vi "input.vi"(8 "error in":errorcluster, 10 "data table in":T1, 11 "io runtime in":refnum<class "io runtime.lvclass">) -> (0 "error out":errorcluster, 2 "data table out":T1, 3 "io runtime out":refnum<class "io runtime.lvclass">)   [LabVIEW 2015, in "io runtime.lvclass"]
doc: "Provides an interface for reading data from a module at runtime. While this interface performs no operations, a child should provide an override which may read from any open sessions, references, or interfaces."
uses:
  io runtime.lvclass
  <vilib>/NI/Tag Bus/table/data table.ctl
  io runtime.lvclass/io runtime.ctl
  FXP I_20_5.ctl
  FXP I_24_5.ctl
  FXP I_24_10.ctl
  <vilib>/NI/Tag Bus/table/data polymorphs/write many/write Doubles.vi
  <vilib>/NI/Tag Bus/table/data polymorphs/write many/write Singles.vi
  <vilib>/NI/Tag Bus/table/data polymorphs/write many/write I64s.vi
  <vilib>/NI/Tag Bus/table/data polymorphs/write many/write I32s.vi
  <vilib>/NI/Tag Bus/table/data polymorphs/write many/write I16s.vi
  <vilib>/NI/Tag Bus/table/data polymorphs/write many/write I8s.vi
  <vilib>/NI/Tag Bus/table/data polymorphs/write many/write U64s.vi
  <vilib>/NI/Tag Bus/table/data polymorphs/write many/write U32s.vi
  <vilib>/NI/Tag Bus/table/data polymorphs/write many/write U16s.vi
  <vilib>/NI/Tag Bus/table/data polymorphs/write many/write U8s.vi
  <vilib>/NI/Tag Bus/table/data polymorphs/write many/write Booleans.vi
  <vilib>/NI/Tag Bus/table/data polymorphs/write one/write Array of Double.vi
  <vilib>/NI/Tag Bus/table/data polymorphs/write one/write Array of Single.vi
  <vilib>/NI/Tag Bus/table/data polymorphs/write one/write Array of I64.vi
  <vilib>/NI/Tag Bus/table/data polymorphs/write one/write Array of I32.vi
  <vilib>/NI/Tag Bus/table/data polymorphs/write one/write Array of I16.vi
  <vilib>/NI/Tag Bus/table/data polymorphs/write one/write Array of I8.vi
  <vilib>/NI/Tag Bus/table/data polymorphs/write one/write Array of U64.vi
  <vilib>/NI/Tag Bus/table/data polymorphs/write one/write Array of U32.vi
  <vilib>/NI/Tag Bus/table/data polymorphs/write one/write Array of U16.vi
  <vilib>/NI/Tag Bus/table/data polymorphs/write one/write Array of U8.vi
  <vilib>/NI/Tag Bus/table/data polymorphs/write one/write Array of Boolean.vi
  <vilib>/rvi/errors/niLvFpgaAdjustHostInterfaceError.vi
  <vilib>/Utility/error.llb/Error Cluster From Error Code.vi
  <vilib>/rvi/interface/nirviReadWriteControl/nirviReadWriteControl.xnode
  <vilib>/rvi/interface/nirviMethod/nirviMethod.xnode
  <vilib>/NI/Tag Bus/table/data table.lvlib
  NiFpgaLv.dll
  <vilib>/rvi/interface/Simulation/niFpgaSimulationCallBeginRW.vi
  <vilib>/FPGAPlugInAG/Dynamic/niLvFpga_ReadFifo_Dynamic.vi
  <vilib>/rvi/errors/niLvFpgaMergeErrorWithErrorCode.vi
panel:
  out "Fails":i32
  out "Elements Remaining":u32
  out "Data":i16[](array[numeric])
  out "Array":u32[](array[numeric])
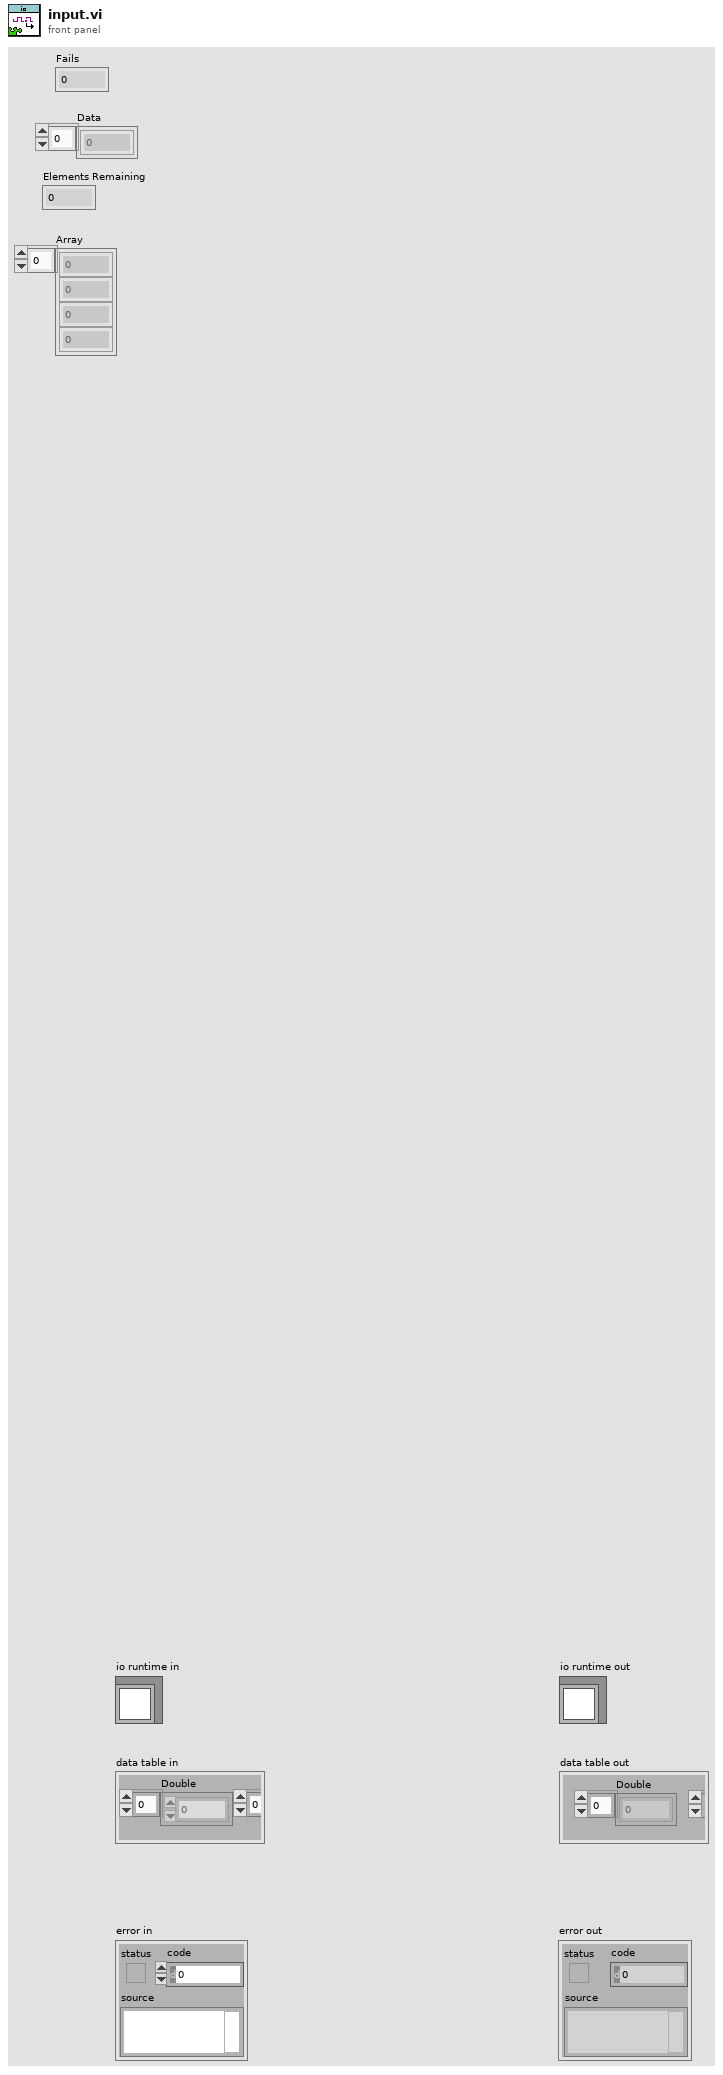
[diagram p1: front panel]
types:
  T1 = typedef "tag bus.lvlib/data table.lvlib/data table.ctl" = cluster{"Double":dbl[], "Single":sgl[], "I64":i64[], "I32":i32[], "I16":i16[], "I8":i8[], "U64":u64[], "U32":u32[], "U16":u16[], "U8":u8[], "Boolean":bool[], "String":string[], "Array of Double":cluster{"DBL Array":dbl[]}[], "Array of Single":cluster{"SGL Array":sgl[]}[], "Array of I64":cluster{"I64 Array":i64[]}[], "Array of I32":cluster{"I32 Array":i32[]}[], "Array of I16":cluster{"I16 Array":i16[]}[], "Array of I8":cluster{"I8 Array":i8[]}[], "Array of U64":cluster{"U64 Array":u64[]}[], "Array of U32":cluster{"U32 Array":u32[]}[], "Array of U16":cluster{"U16 Array":u16[]}[], "Array of U8":cluster{"U8 Array":u8[]}[], "Array of Boolean":cluster{"Boolean Array":bool[]}[], "Array of String":cluster{"String Array":string[]}[]}
  T2 = typedef "io runtime.lvclass/control index set.ctl" = cluster{"data type":T3, "fpga res type":T4[], "fpga resource":refnum<k20>[], "data indexes":i32[], "fifo timeout":refnum<k20>[], "fifo reset":refnum<k20>[], "fifo average":i32[], "fifo samples":u32[], "fifo channels":u32[]}
  T3 = typedef "tag bus.lvlib/tag descriptor.lvclass/Data Type.ctl" = enum16{"Double", "Single", "I64", "I32", "I16", "I8", "U64", "U32", "U16", "U8", "Boolean", "String", "Array of Double", "Array of Single", "Array of I64", "Array of I32", "Array of I16", "Array of I8", "Array of U64", "Array of U32", "Array of U16", "Array of U8", "Array of Boolean", "Array of String"}
  T4 = typedef "io configuration.lvclass/fpga resource supported data types.ctl" = enum16{"Invalid Type", "Single", "I64", "I32", "I16", "I8", "U64", "U32", "U16", "U8", "Boolean", "FXP I,20,5", "FXP I,24,5", "FXP I,24,10", "Fifo 1023,I16"}
  T5 = typedef "io runtime.lvclass/FXP I_20_5.ctl" = refnum<k20>
  T6 = typedef "io runtime.lvclass/FXP I_24_5.ctl" = refnum<k20>
  T7 = typedef "io runtime.lvclass/FXP I_24_10.ctl" = refnum<k20>
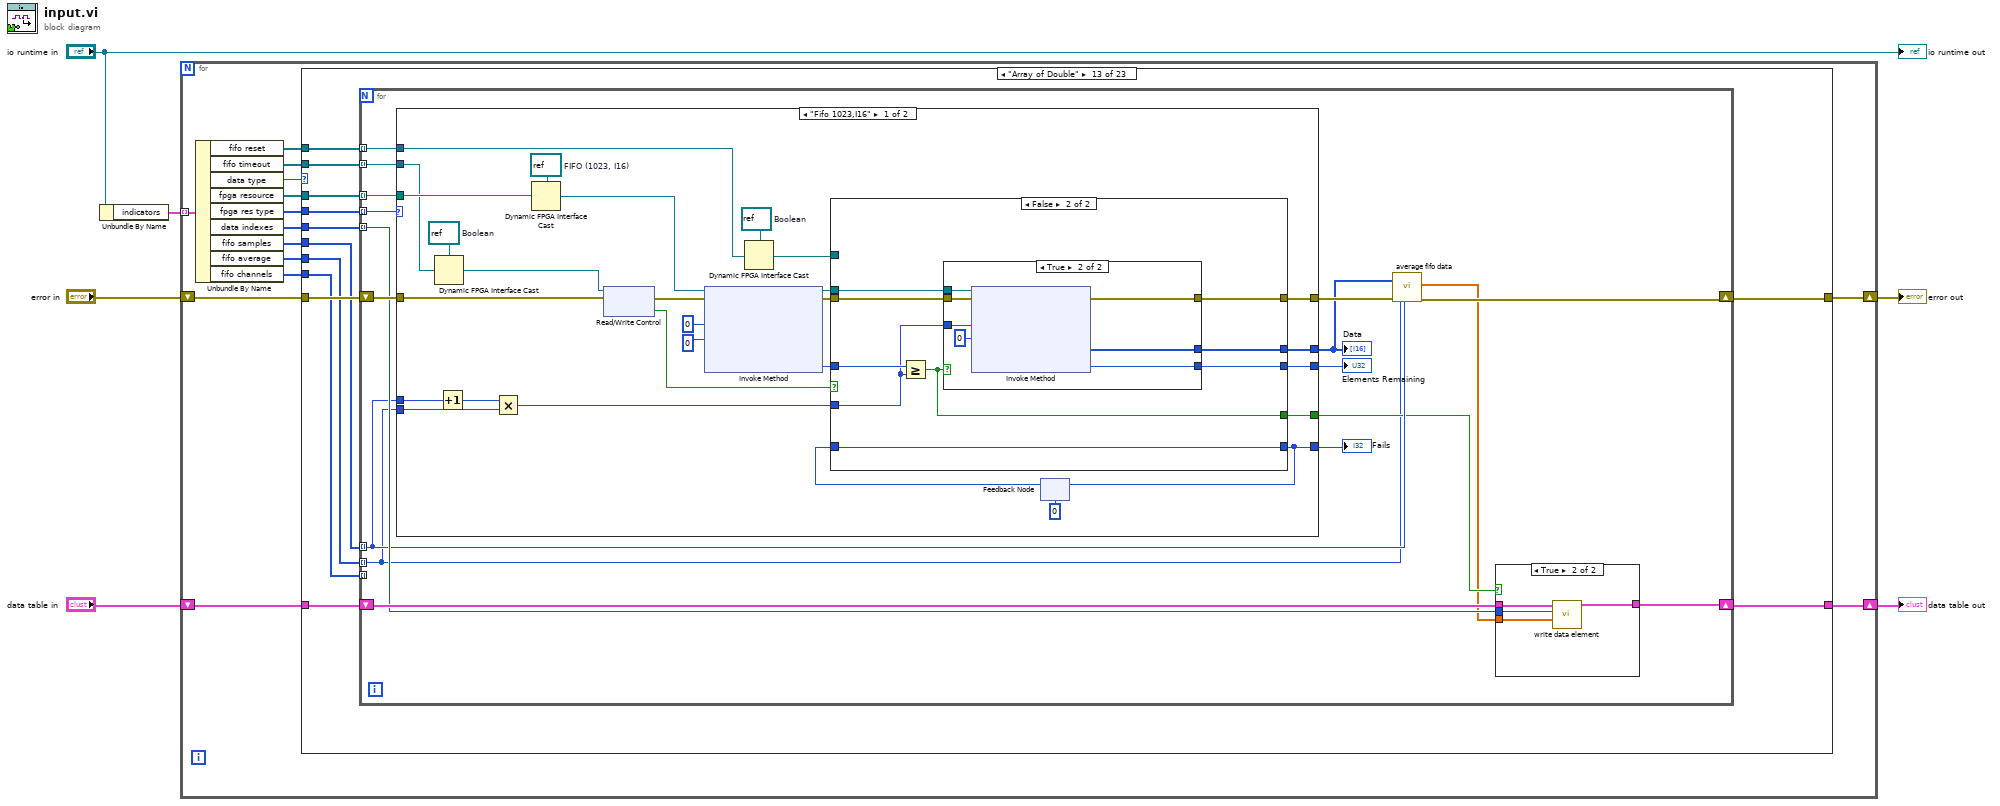
[diagram p0: block diagram]
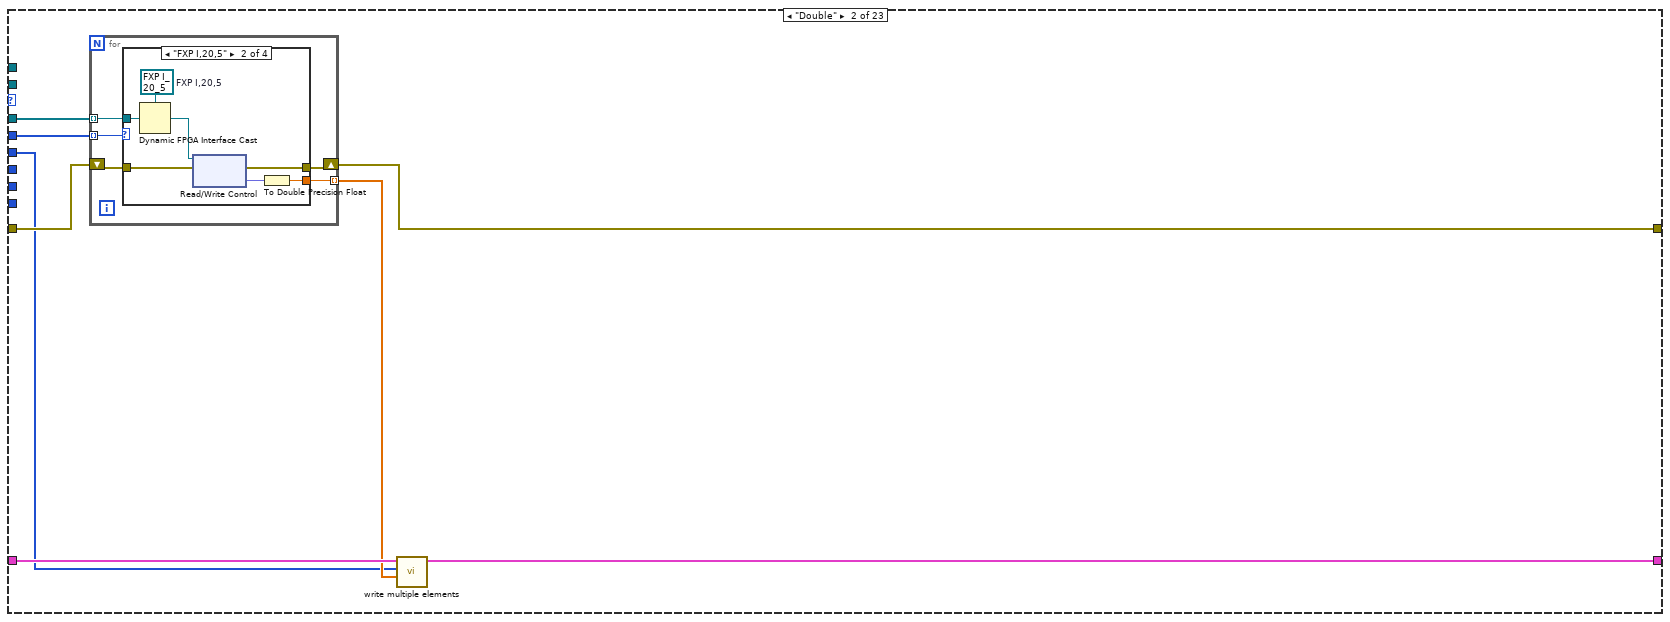
[diagram p3: hidden frame]
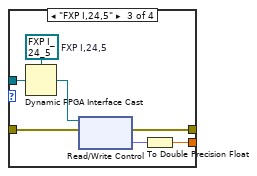
[diagram p5: hidden frame]
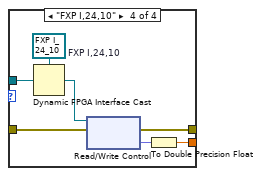
[diagram p6: hidden frame]
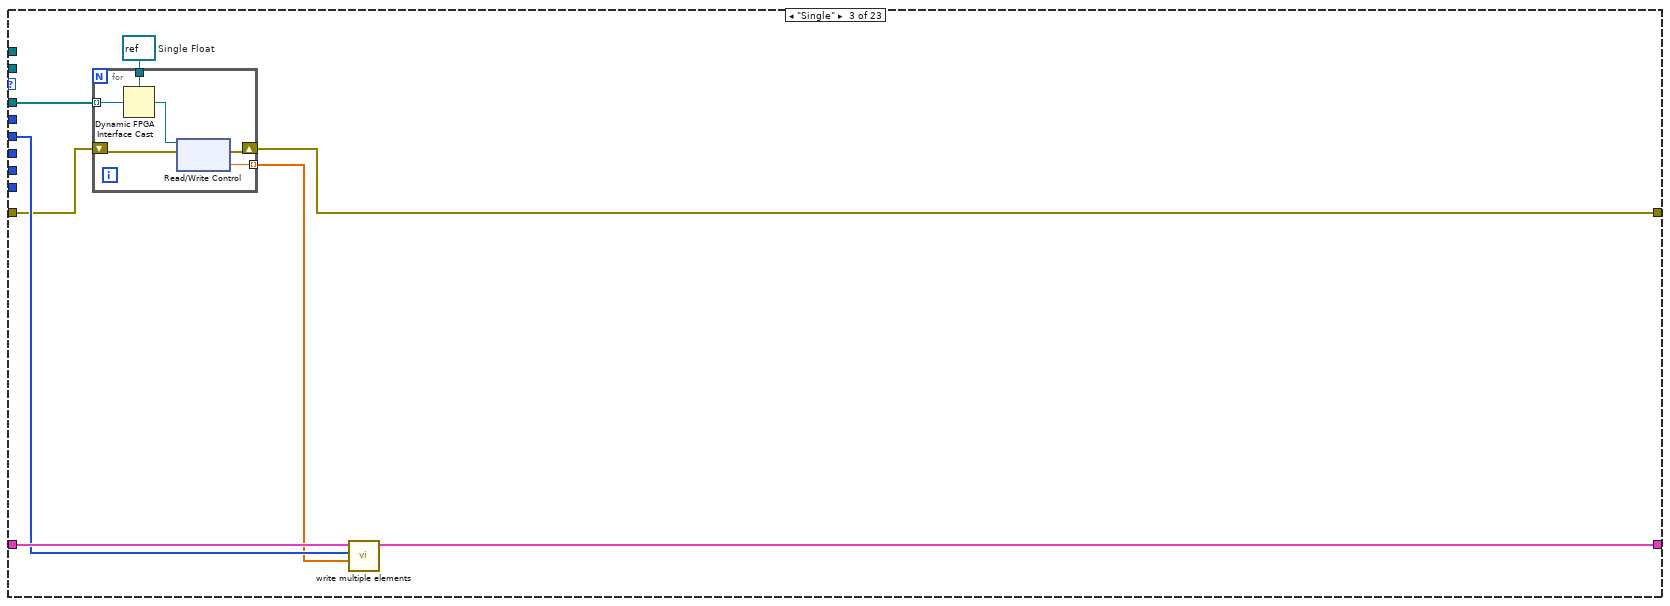
[diagram p7: hidden frame]
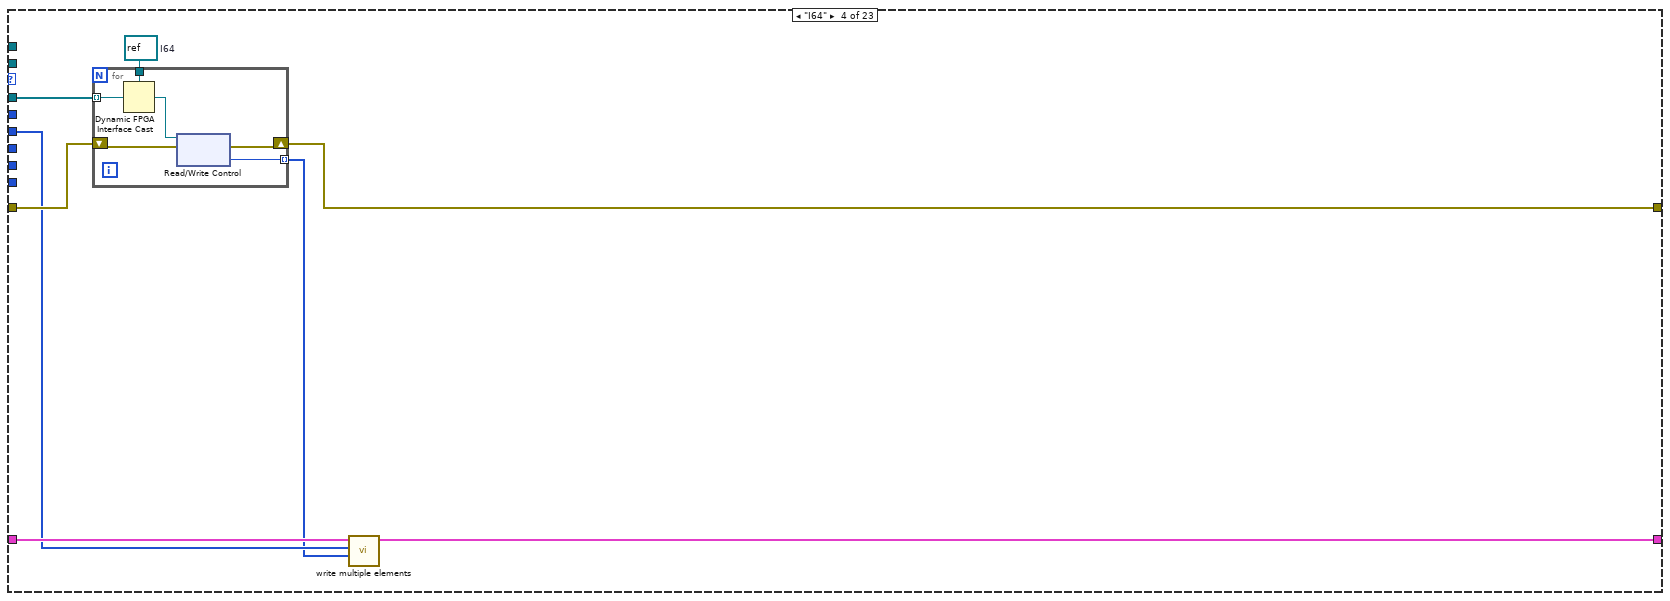
[diagram p8: hidden frame]
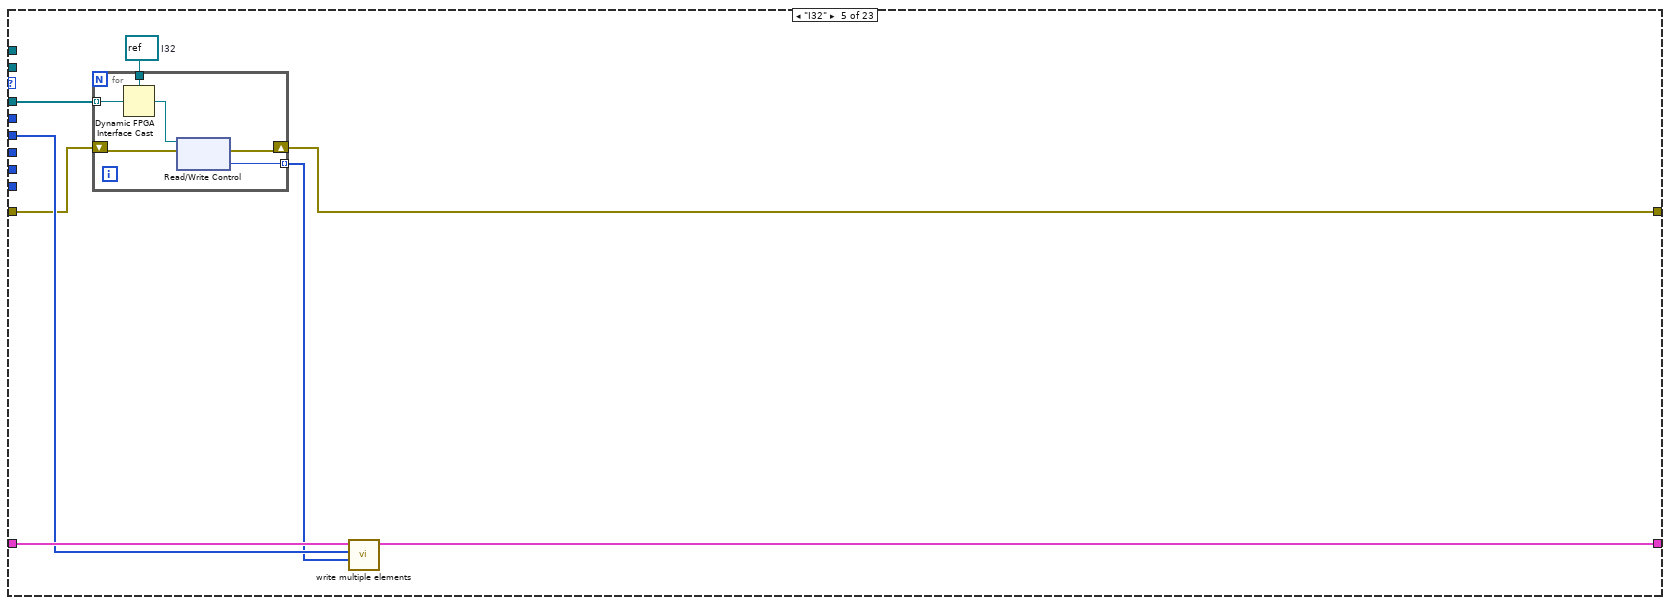
[diagram p9: hidden frame]
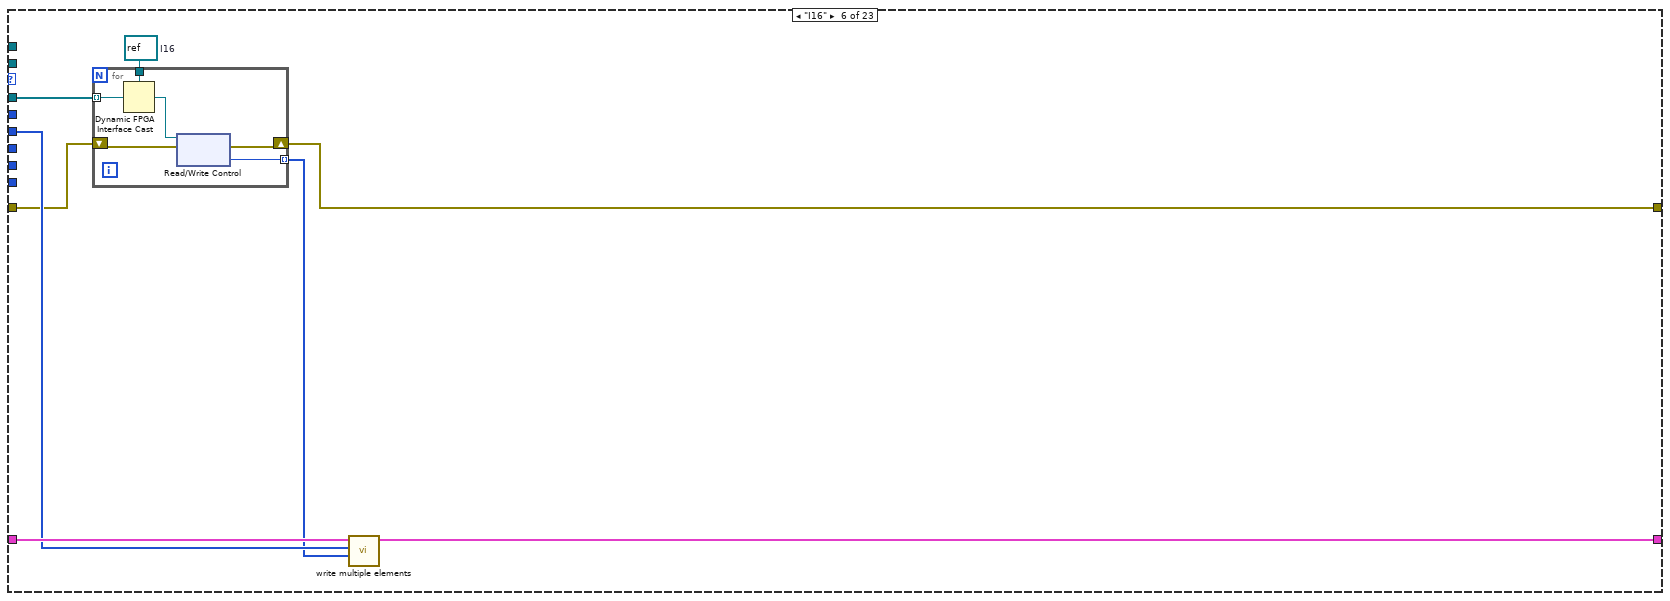
[diagram p10: hidden frame]
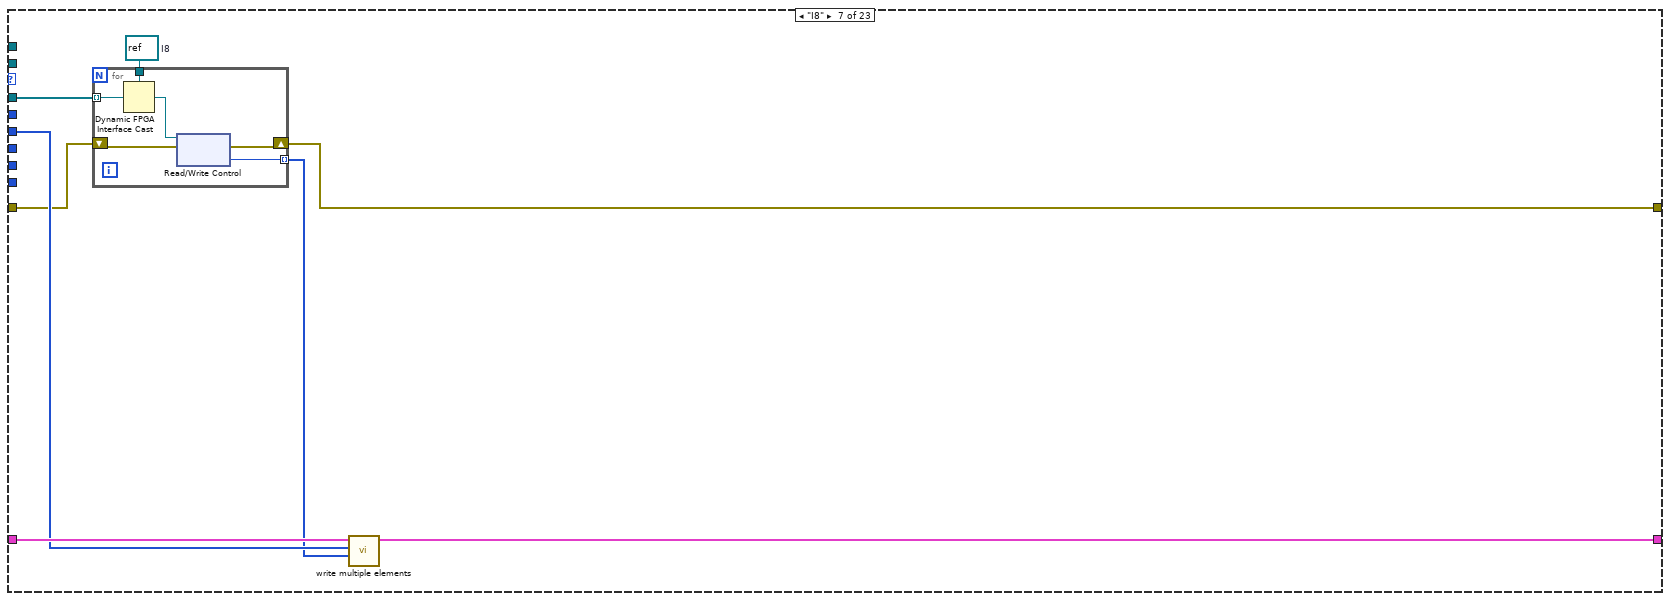
[diagram p11: hidden frame]
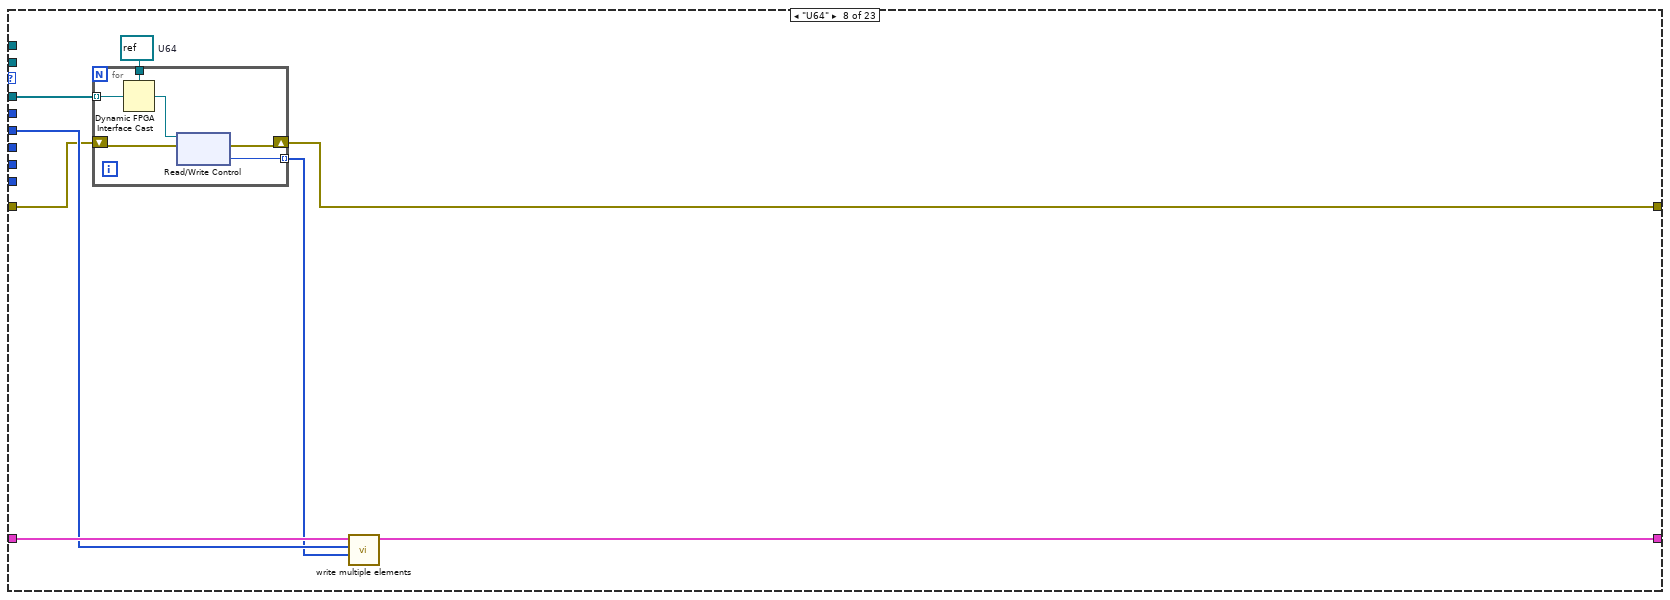
[diagram p12: hidden frame]
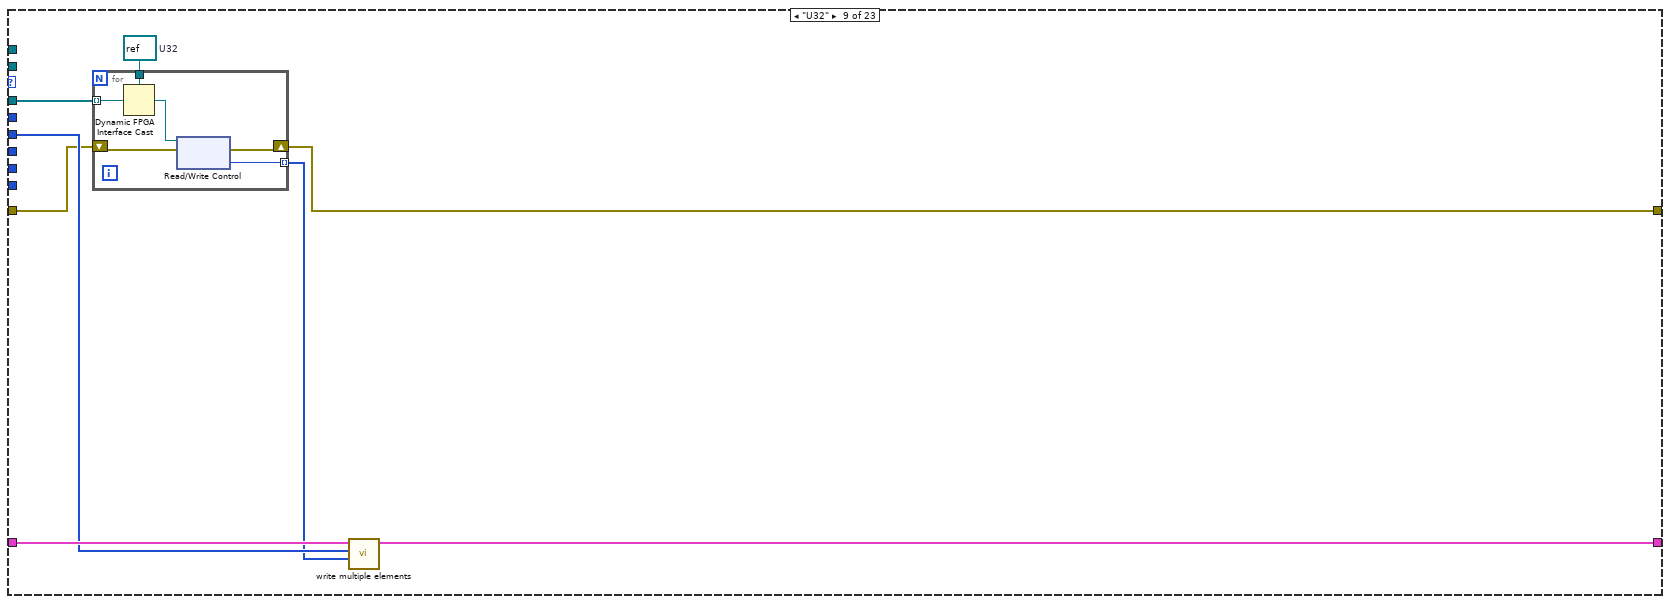
[diagram p13: hidden frame]
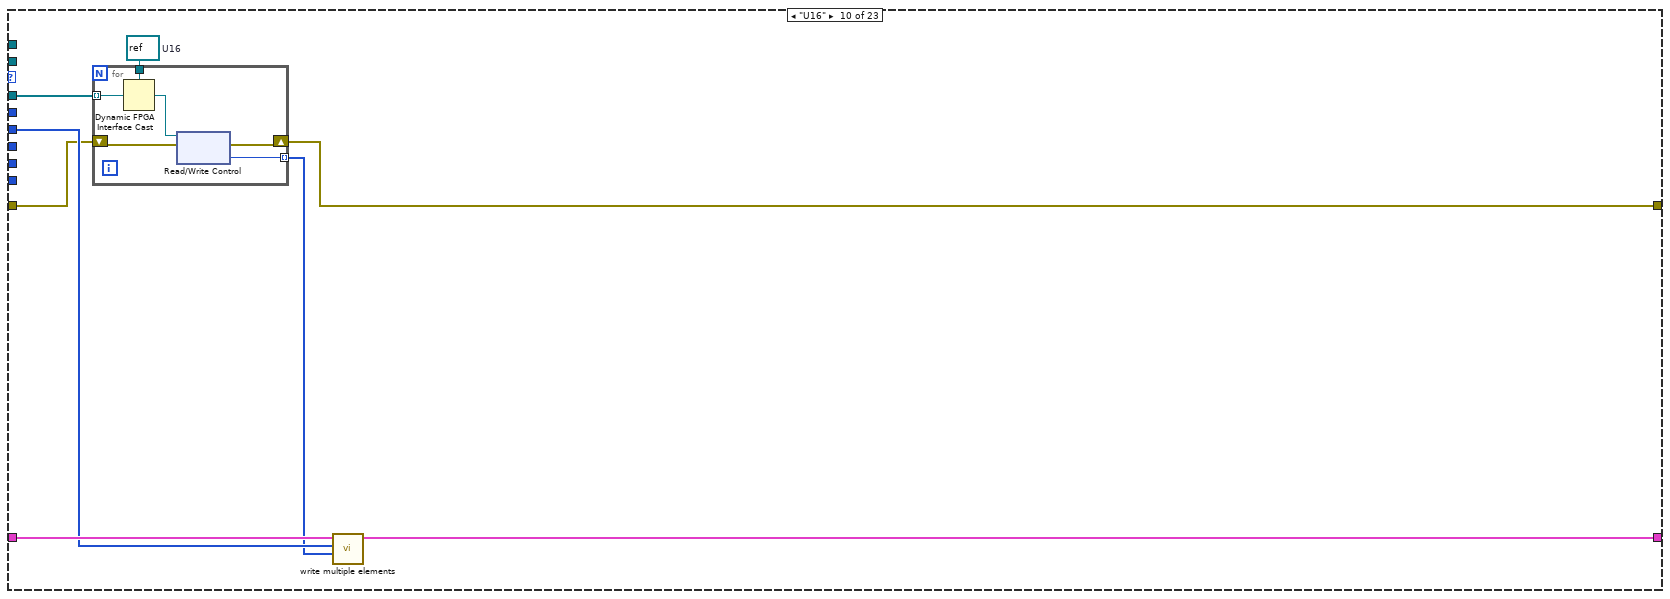
[diagram p14: hidden frame]
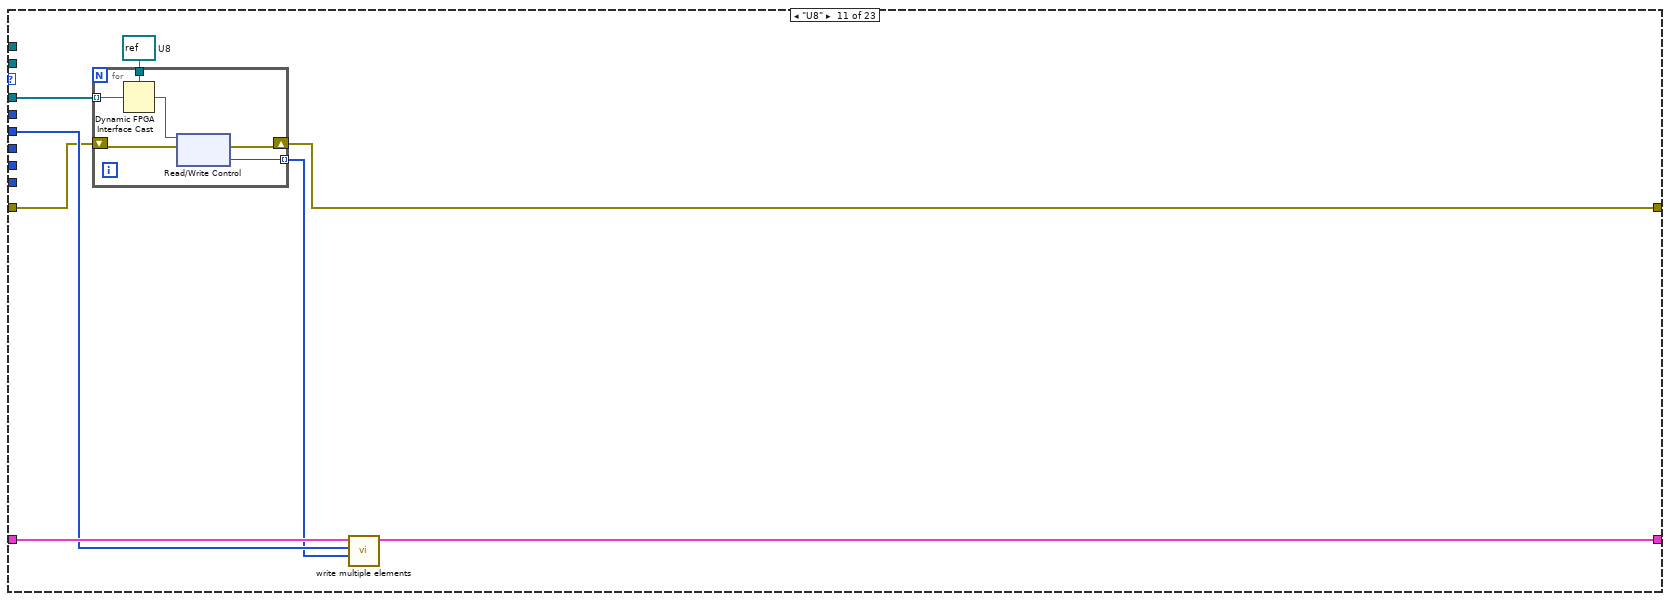
[diagram p15: hidden frame]
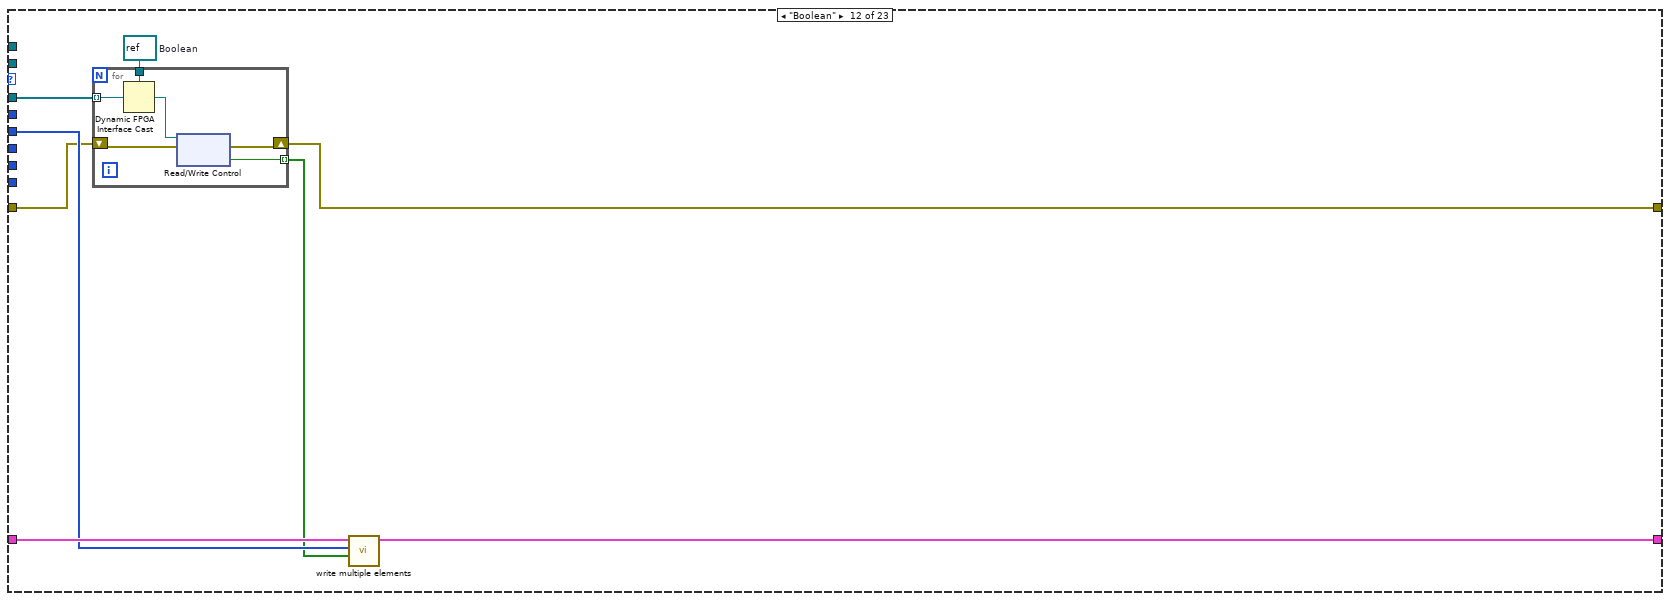
[diagram p16: hidden frame]
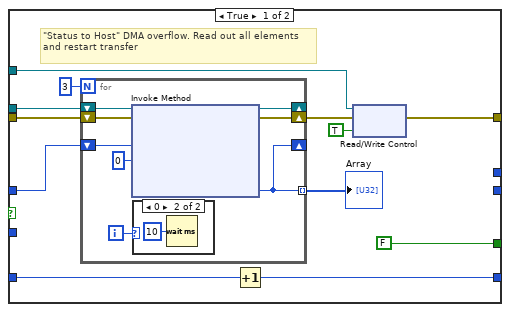
[diagram p18: hidden frame]
diagram:
  n1 = Unbundle By Name("io runtime in") -> ("indicators"=w1:T2[])
  n2 = for {
    shift-right: [w17] -> w3
    shift-left: "data table in" -> [w18]
    shift-right: [w16] -> w4
    shift-left: "error in" -> [w15]
    tunnel: w1 -> [w20] mode=indexing
    n3 = Unbundle By Name(w20) -> ("fifo reset"=w11:refnum<k20>[], "fifo timeout"=w10:refnum<k20>[], "data type"=w19:T3, "fpga resource"=w14:refnum<k20>[], "fpga res type"=w12:T4[], "data indexes"=w13:i32[], "fifo samples"=w8:u32[], "fifo average"=w9:i32[], "fifo channels"=w7:u32[])
    n4 = case shown="\"Array of Double\"" w19 {
      tunnel: w13 -> [_ w23 w63 w76 w91 w105 w119 w133 w147 w161 w175 w189 w200 w302 w317 w332 w347 w362 w377 w392 w407 w422 w437]
      tunnel: w15 -> [w22 w27 w61 w79 w89 w103 w117 w131 w145 w159 w173 w187 w209 w301 w316 w331 w346 w361 w376 w391 w406 w421 w436]
      tunnel: w18 -> [w21 w30 w65 w78 w93 w107 w121 w135 w149 w163 w177 w191 w201 w304 w319 w334 w349 w364 w379 w394 w409 w424 w439]
      tunnel: [w21 w29 w64 w77 w92 w106 w120 w134 w148 w162 w176 w190 w199 w303 w318 w333 w348 w363 w378 w393 w408 w423 w438] -> w17
      tunnel: [w22 w26 w60 w74 w88 w102 w116 w130 w144 w158 w172 w186 w207 w300 w315 w330 w345 w360 w375 w390 w405 w420 w435] -> w16
      tunnel: w14 -> [_ w28 w62 w75 w90 w104 w118 w132 w146 w160 w174 w188 w208 w299 w314 w329 w344 w359 w374 w389 w404 w419 w434]
      tunnel: w12 -> [_ w25 _ _ _ _ _ _ _ _ _ _ w206 _ _ _ _ _ _ _ _ _ _]
      tunnel: w11 -> [_ _ _ _ _ _ _ _ _ _ _ _ w205 _ _ _ _ _ _ _ _ _ _]
      tunnel: w10 -> [_ _ _ _ _ _ _ _ _ _ _ _ w204 _ _ _ _ _ _ _ _ _ _]
      tunnel: w9 -> [_ _ _ _ _ _ _ _ _ _ _ _ w202 _ _ _ _ _ _ _ _ _ _]
      tunnel: w8 -> [_ _ _ _ _ _ _ _ _ _ _ _ w203 _ _ _ _ _ _ _ _ _ _]
      tunnel: w7 -> [_ _ _ _ _ _ _ _ _ _ _ _ w198 _ _ _ _ _ _ _ _ _ _]
      frame Default {
      }
      frame "Double" {
        n5 = for {
          tunnel: w28 -> [w35] mode=indexing
          shift-right: [w33] -> w26
          shift-left: w27 -> [w34]
          tunnel: [w32] -> w24 mode=indexing
          tunnel: w25 -> [w31] mode=indexing
          n6 = case shown="\"FXP I,20,5\"" w31 {
            tunnel: w35 -> [_ w43 w50 w57]
            tunnel: w34 -> [w36 w42 w49 w56]
            tunnel: [w36 w41 w48 w55] -> w33
            tunnel: [_ w38 w45 w52] -> w32
            frame "Invalid Type", Default {
            }
            frame "FXP I,20,5" {
              w40 = T5 refnum  # FXP I,20,5
              n7 = Dynamic FPGA Interface Cast(Session In=w40, Type=w43) -> (Session Out=w37:T5)
              n8 = xnode "Read/Write Control"("FPGA VI Reference In"=w37, "error in"=w42) -> ("error out"=w41:errorcluster, "Value"=w39:fxp<+/-,20,5>)  [unwired: 1 out]
              n9 = To Double Precision Float(number=w39) -> (double precision float=w38:dbl)
            }
            frame "FXP I,24,5" {
              w47 = T6 refnum  # FXP I,24,5
              n10 = Dynamic FPGA Interface Cast(Session In=w47, Type=w50) -> (Session Out=w44:T6)
              n11 = xnode "Read/Write Control"("FPGA VI Reference In"=w44, "error in"=w49) -> ("error out"=w48:errorcluster, "Value"=w46:fxp<+/-,24,5>)  [unwired: 1 out]
              n12 = To Double Precision Float(number=w46) -> (double precision float=w45:dbl)
            }
            frame "FXP I,24,10" {
              w54 = T7 refnum  # FXP I,24,10
              n13 = Dynamic FPGA Interface Cast(Session In=w54, Type=w57) -> (Session Out=w51:T7)
              n14 = xnode "Read/Write Control"("FPGA VI Reference In"=w51, "error in"=w56) -> ("error out"=w55:errorcluster, "Value"=w53:fxp<+/-,24,10>)  [unwired: 1 out]
              n15 = To Double Precision Float(number=w53) -> (double precision float=w52:dbl)
            }
          }
        }
        n16 = call-poly <vilib>:"write multiple elements.vi"("values"=w24, "indices"=w23, "data table in"=w30) -> ("data table out"=w29:T1)  [unwired: 8 in]
      }
      frame "Single" {
        w59 = refnum<k20> refnum  # Single Float
        n17 = for {
          tunnel: w62 -> [w71] mode=indexing
          shift-right: [w68] -> w60
          shift-left: w61 -> [w69]
          tunnel: [w67] -> w58 mode=indexing
          tunnel: w59 -> [w66]
          n18 = Dynamic FPGA Interface Cast(Session In=w66, Type=w71) -> (Session Out=w70:refnum<k20>)
          n19 = xnode "Read/Write Control"("FPGA VI Reference In"=w70, "error in"=w69) -> ("error out"=w68:errorcluster, "Value"=w67:sgl)  [unwired: 1 out]
        }
        n20 = call-poly <vilib>:"write multiple elements.vi"("values"=w58, "indices"=w63, "data table in"=w65) -> ("data table out"=w64:T1)  [unwired: 8 in]
      }
      frame "I64" {
        w72 = refnum<k20> refnum  # I64
        n21 = for {
          tunnel: w75 -> [w85] mode=indexing
          shift-right: [w82] -> w74
          shift-left: w79 -> [w83]
          tunnel: [w81] -> w73 mode=indexing
          tunnel: w72 -> [w80]
          n22 = Dynamic FPGA Interface Cast(Session In=w80, Type=w85) -> (Session Out=w84:refnum<k20>)
          n23 = xnode "Read/Write Control"("FPGA VI Reference In"=w84, "error in"=w83) -> ("error out"=w82:errorcluster, "Value"=w81:i64)  [unwired: 1 out]
        }
        n24 = call-poly <vilib>:"write multiple elements.vi"("values"=w73, "indices"=w76, "data table in"=w78) -> ("data table out"=w77:T1)  [unwired: 8 in]
      }
      frame "I32" {
        w86 = refnum<k20> refnum  # I32
        n25 = for {
          tunnel: w90 -> [w99] mode=indexing
          shift-right: [w96] -> w88
          shift-left: w89 -> [w97]
          tunnel: [w95] -> w87 mode=indexing
          tunnel: w86 -> [w94]
          n26 = Dynamic FPGA Interface Cast(Session In=w94, Type=w99) -> (Session Out=w98:refnum<k20>)
          n27 = xnode "Read/Write Control"("FPGA VI Reference In"=w98, "error in"=w97) -> ("error out"=w96:errorcluster, "Value"=w95:i32)  [unwired: 1 out]
        }
        n28 = call-poly <vilib>:"write multiple elements.vi"("values"=w87, "indices"=w91, "data table in"=w93) -> ("data table out"=w92:T1)  [unwired: 8 in]
      }
      frame "I16" {
        w100 = refnum<k20> refnum  # I16
        n29 = for {
          tunnel: w104 -> [w113] mode=indexing
          shift-right: [w110] -> w102
          shift-left: w103 -> [w111]
          tunnel: [w109] -> w101 mode=indexing
          tunnel: w100 -> [w108]
          n30 = Dynamic FPGA Interface Cast(Session In=w108, Type=w113) -> (Session Out=w112:refnum<k20>)
          n31 = xnode "Read/Write Control"("FPGA VI Reference In"=w112, "error in"=w111) -> ("error out"=w110:errorcluster, "Value"=w109:i16)  [unwired: 1 out]
        }
        n32 = call-poly <vilib>:"write multiple elements.vi"("values"=w101, "indices"=w105, "data table in"=w107) -> ("data table out"=w106:T1)  [unwired: 8 in]
      }
      frame "I8" {
        w114 = refnum<k20> refnum  # I8
        n33 = for {
          tunnel: w118 -> [w127] mode=indexing
          shift-right: [w124] -> w116
          shift-left: w117 -> [w125]
          tunnel: [w123] -> w115 mode=indexing
          tunnel: w114 -> [w122]
          n34 = Dynamic FPGA Interface Cast(Session In=w122, Type=w127) -> (Session Out=w126:refnum<k20>)
          n35 = xnode "Read/Write Control"("FPGA VI Reference In"=w126, "error in"=w125) -> ("error out"=w124:errorcluster, "Value"=w123:i8)  [unwired: 1 out]
        }
        n36 = call-poly <vilib>:"write multiple elements.vi"("values"=w115, "indices"=w119, "data table in"=w121) -> ("data table out"=w120:T1)  [unwired: 8 in]
      }
      frame "U64" {
        w128 = refnum<k20> refnum  # U64
        n37 = for {
          tunnel: w132 -> [w141] mode=indexing
          shift-right: [w138] -> w130
          shift-left: w131 -> [w139]
          tunnel: [w137] -> w129 mode=indexing
          tunnel: w128 -> [w136]
          n38 = Dynamic FPGA Interface Cast(Session In=w136, Type=w141) -> (Session Out=w140:refnum<k20>)
          n39 = xnode "Read/Write Control"("FPGA VI Reference In"=w140, "error in"=w139) -> ("error out"=w138:errorcluster, "Value"=w137:u64)  [unwired: 1 out]
        }
        n40 = call-poly <vilib>:"write multiple elements.vi"("values"=w129, "indices"=w133, "data table in"=w135) -> ("data table out"=w134:T1)  [unwired: 8 in]
      }
      frame "U32" {
        w142 = refnum<k20> refnum  # U32
        n41 = for {
          tunnel: w146 -> [w155] mode=indexing
          shift-right: [w152] -> w144
          shift-left: w145 -> [w153]
          tunnel: [w151] -> w143 mode=indexing
          tunnel: w142 -> [w150]
          n42 = Dynamic FPGA Interface Cast(Session In=w150, Type=w155) -> (Session Out=w154:refnum<k20>)
          n43 = xnode "Read/Write Control"("FPGA VI Reference In"=w154, "error in"=w153) -> ("error out"=w152:errorcluster, "Value"=w151:u32)  [unwired: 1 out]
        }
        n44 = call-poly <vilib>:"write multiple elements.vi"("values"=w143, "indices"=w147, "data table in"=w149) -> ("data table out"=w148:T1)  [unwired: 8 in]
      }
      frame "U16" {
        w156 = refnum<k20> refnum  # U16
        n45 = for {
          tunnel: w160 -> [w169] mode=indexing
          shift-right: [w166] -> w158
          shift-left: w159 -> [w167]
          tunnel: [w165] -> w157 mode=indexing
          tunnel: w156 -> [w164]
          n46 = Dynamic FPGA Interface Cast(Session In=w164, Type=w169) -> (Session Out=w168:refnum<k20>)
          n47 = xnode "Read/Write Control"("FPGA VI Reference In"=w168, "error in"=w167) -> ("error out"=w166:errorcluster, "Value"=w165:u16)  [unwired: 1 out]
        }
        n48 = call-poly <vilib>:"write multiple elements.vi"("values"=w157, "indices"=w161, "data table in"=w163) -> ("data table out"=w162:T1)  [unwired: 8 in]
      }
      frame "U8" {
        w170 = refnum<k20> refnum  # U8
        n49 = for {
          tunnel: w174 -> [w183] mode=indexing
          shift-right: [w180] -> w172
          shift-left: w173 -> [w181]
          tunnel: [w179] -> w171 mode=indexing
          tunnel: w170 -> [w178]
          n50 = Dynamic FPGA Interface Cast(Session In=w178, Type=w183) -> (Session Out=w182:refnum<k20>)
          n51 = xnode "Read/Write Control"("FPGA VI Reference In"=w182, "error in"=w181) -> ("error out"=w180:errorcluster, "Value"=w179:u8)  [unwired: 1 out]
        }
        n52 = call-poly <vilib>:"write multiple elements.vi"("values"=w171, "indices"=w175, "data table in"=w177) -> ("data table out"=w176:T1)  [unwired: 8 in]
      }
      frame "Boolean" {
        w184 = refnum<k20> refnum  # Boolean
        n53 = for {
          tunnel: w188 -> [w197] mode=indexing
          shift-right: [w194] -> w186
          shift-left: w187 -> [w195]
          tunnel: [w193] -> w185 mode=indexing
          tunnel: w184 -> [w192]
          n54 = Dynamic FPGA Interface Cast(Session In=w192, Type=w197) -> (Session Out=w196:refnum<k20>)
          n55 = xnode "Read/Write Control"("FPGA VI Reference In"=w196, "error in"=w195) -> ("error out"=w194:errorcluster, "Value"=w193:bool)  [unwired: 1 out]
        }
        n56 = call-poly <vilib>:"write multiple elements.vi"("values"=w185, "indices"=w189, "data table in"=w191) -> ("data table out"=w190:T1)  [unwired: 8 in]
      }
      frame "Array of Double" {
        n57 = for {
          tunnel: w208 -> [w225] mode=indexing
          shift-right: [w215] -> w207
          shift-left: w209 -> [w224]
          tunnel: w203 -> [w213] mode=indexing
          tunnel: w206 -> [w223] mode=indexing
          tunnel: w205 -> [w222] mode=indexing
          tunnel: w204 -> [w221] mode=indexing
          tunnel: w202 -> [w211] mode=indexing
          tunnel: w200 -> [w218] mode=indexing
          shift-right: [w217] -> w199
          shift-left: w201 -> [w219]
          tunnel: w198 -> [_] mode=indexing
          n58 = case shown="\"Fifo 1023,I16\"" w223 {
            tunnel: [w235 w298] -> w216
            tunnel: [w236 _] -> w214
            tunnel: [w254 _] -> w226
            tunnel: [w253 _] -> w212
            tunnel: [w249 _] -> w220
            tunnel: w225 -> [w246 _]
            tunnel: w213 -> [w244 _]
            tunnel: w224 -> [w243 w298]
            tunnel: w222 -> [w241 _]
            tunnel: w221 -> [w238 _]
            tunnel: w211 -> [w232 _]
            frame "Fifo 1023,I16" {
              w239 = refnum<k20> refnum  # Boolean
              w242 = refnum<k20> refnum  # Boolean
              w247 = refnum<k20> refnum  # FIFO (1023, I16)
              n59 = Dynamic FPGA Interface Cast(Session In=w239, Type=w238) -> (Session Out=w237:refnum<k20>)
              n60 = Increment(x=w244) -> (x+1=w234:u32)
              n61 = Multiply(x=w234, y=w232) -> (x*y=w233:u32)
              n62 = Dynamic FPGA Interface Cast(Session In=w247, Type=w246) -> (Session Out=w245:refnum<k20>)
              n63 = xnode "Read/Write Control"("FPGA VI Reference In"=w237, "error in"=w243) -> ("error out"=w259:errorcluster, "Value"=w248:bool)  [unwired: 1 out]
              n64 = xnode "Invoke Method"("FPGA VI Reference In"=w245, "error in"=w259, "Number of Elements"=u32 0, "Timeout (ms)"=0) -> ("FPGA VI Reference Out"=w257:refnum<k20>, "error out"=w256:errorcluster, "Elements Remaining"=w255:u32)  [unwired: 1 out]
              n65 = Dynamic FPGA Interface Cast(Session In=w242, Type=w241) -> (Session Out=w240:refnum<k20>)
              n66 = feedback #1(0) -> (w250:i32)
              n67 = case shown="False" w248 {
                tunnel: w257 -> [w271 w289]
                tunnel: w256 -> [w270 w288]
                tunnel: w255 -> [w263 w287]
                tunnel: [w266 w281] -> w235
                tunnel: w233 -> [_ w283]
                tunnel: [_ w282] -> w236
                tunnel: [_ w286] -> w254
                tunnel: [FALSE w285] -> w253
                tunnel: [w265 w284] -> w249
                tunnel: w250 -> [w264 w284]
                tunnel: w240 -> [w260 _]
                frame True {
                  # "\"Status to Host\" DMA overflow. Read out all elements and restart transfer"
                  n68 = for {
                    N: 3 -> [_]
                    shift-right: [w276] -> _
                    shift-left: w271 -> [w279]
                    shift-right: [w277] -> w269
                    shift-left: w270 -> [w278]
                    shift-right: [w273] -> _
                    shift-left: w263 -> [w274]
                    tunnel: [w273] -> w261 mode=indexing
                    i -> [w272]
                    n69 = xnode "Invoke Method"("FPGA VI Reference In"=w279, "error in"=w278, "Number of Elements"=w274, "Timeout (ms)"=0) -> ("FPGA VI Reference Out"=w276:refnum<k20>, "error out"=w277:errorcluster, "Elements Remaining"=w273:u32)  [unwired: 1 out]
                    n70 = case shown="0" w272 {
                      frame 1, Default {
                      }
                      frame 0 {
                        n71 = Wait (ms)(milliseconds to wait=u32 10) -> ()  [unwired: 1 out]
                      }
                    }
                  }
                  "Array" <- w261
                  n72 = Increment(x=w264) -> (x+1=w265:i32)
                  n73 = xnode "Read/Write Control"("FPGA VI Reference In"=w260, "error in"=w269, "Value"=TRUE ("T to H Reset")) -> ("error out"=w266:errorcluster)  [unwired: 1 out]
                }
                frame False {
                  n74 = Greater Or Equal?(x=w287, y=w283) -> (x >= y?=w285:bool)
                  n75 = case shown="True" w285 {
                    tunnel: w289 -> [_ w297]
                    tunnel: w288 -> [w290 w296]
                    tunnel: [w290 w294] -> w281
                    tunnel: w283 -> [_ w293]
                    tunnel: [_ w292] -> w282
                    tunnel: [_ w291] -> w286
                    frame False {
                    }
                    frame True {
                      n76 = xnode "Invoke Method"("FPGA VI Reference In"=w297, "error in"=w296, "Number of Elements"=w293, "Timeout (ms)"=0) -> ("error out"=w294:errorcluster, "Data"=w292:i16[], "Elements Remaining"=w291:u32)  [unwired: 1 out]
                    }
                  }
                }
              }
              n77 = feedback-in #1(w249) -> ()
            }
            frame Default {
            }
          }
          "Data" <- w214
          "Elements Remaining" <- w226
          "Fails" <- w220
          n78 = call "average fifo data.vi"("Interleaved Data"=w214, "Samples"=w213, "Acc"=w211, "error in (no error)"=w216) -> ("Avg Scan"=w210:dbl[], "error out (no error)"=w215:errorcluster)  [unwired: 13 in, 1 out]
          n79 = case shown="True" w212 {
            tunnel: w219 -> [w227 w231]
            tunnel: w218 -> [_ w230]
            tunnel: [w227 w229] -> w217
            tunnel: w210 -> [_ w228]
            frame False {
            }
            frame True {
              n80 = call-poly <vilib>:"write data element.vi"("value"=w228, "index"=w230, "data table in"=w231) -> ("data table out"=w229:T1)  [unwired: 8 in]
            }
          }
        }
      }
      frame "Array of Single" {
        n81 = for {
          tunnel: w302 -> [w311] mode=indexing
          shift-right: [w308] -> w300
          shift-left: w301 -> [w307]
          shift-right: [w312] -> w303
          shift-left: w304 -> [w313]
          tunnel: w299 -> [w309] mode=indexing
          w306 = refnum<k20> refnum  # Array Single
          n82 = Dynamic FPGA Interface Cast(Session In=w306, Type=w309) -> (Session Out=w310:refnum<k20>)
          n83 = xnode "Read/Write Control"("FPGA VI Reference In"=w310, "error in"=w307) -> ("error out"=w308:errorcluster, "Value"=w305:sgl[])  [unwired: 1 out]
          n84 = call-poly <vilib>:"write data element.vi"("value"=w305, "index"=w311, "data table in"=w313) -> ("data table out"=w312:T1)  [unwired: 8 in]
        }
      }
      frame "Array of I64" {
        n85 = for {
          tunnel: w317 -> [w326] mode=indexing
          shift-right: [w323] -> w315
          shift-left: w316 -> [w322]
          shift-right: [w327] -> w318
          shift-left: w319 -> [w328]
          tunnel: w314 -> [w324] mode=indexing
          w320 = refnum<k20> refnum  # Array I64
          n86 = Dynamic FPGA Interface Cast(Session In=w320, Type=w324) -> (Session Out=w325:refnum<k20>)
          n87 = xnode "Read/Write Control"("FPGA VI Reference In"=w325, "error in"=w322) -> ("error out"=w323:errorcluster, "Value"=w321:i64[])  [unwired: 1 out]
          n88 = call-poly <vilib>:"write data element.vi"("value"=w321, "index"=w326, "data table in"=w328) -> ("data table out"=w327:T1)  [unwired: 8 in]
        }
      }
      frame "Array of I32" {
        n89 = for {
          tunnel: w332 -> [w341] mode=indexing
          shift-right: [w338] -> w330
          shift-left: w331 -> [w337]
          shift-right: [w342] -> w333
          shift-left: w334 -> [w343]
          tunnel: w329 -> [w339] mode=indexing
          w335 = refnum<k20> refnum  # Array I32
          n90 = Dynamic FPGA Interface Cast(Session In=w335, Type=w339) -> (Session Out=w340:refnum<k20>)
          n91 = xnode "Read/Write Control"("FPGA VI Reference In"=w340, "error in"=w337) -> ("error out"=w338:errorcluster, "Value"=w336:i32[])  [unwired: 1 out]
          n92 = call-poly <vilib>:"write data element.vi"("value"=w336, "index"=w341, "data table in"=w343) -> ("data table out"=w342:T1)  [unwired: 8 in]
        }
      }
      frame "Array of I16" {
        n93 = for {
          tunnel: w347 -> [w356] mode=indexing
          shift-right: [w353] -> w345
          shift-left: w346 -> [w352]
          shift-right: [w357] -> w348
          shift-left: w349 -> [w358]
          tunnel: w344 -> [w354] mode=indexing
          w350 = refnum<k20> refnum  # Array I16
          n94 = Dynamic FPGA Interface Cast(Session In=w350, Type=w354) -> (Session Out=w355:refnum<k20>)
          n95 = xnode "Read/Write Control"("FPGA VI Reference In"=w355, "error in"=w352) -> ("error out"=w353:errorcluster, "Value"=w351:i16[])  [unwired: 1 out]
          n96 = call-poly <vilib>:"write data element.vi"("value"=w351, "index"=w356, "data table in"=w358) -> ("data table out"=w357:T1)  [unwired: 8 in]
        }
      }
      frame "Array of I8" {
        n97 = for {
          tunnel: w362 -> [w371] mode=indexing
          shift-right: [w368] -> w360
          shift-left: w361 -> [w367]
          shift-right: [w372] -> w363
          shift-left: w364 -> [w373]
          tunnel: w359 -> [w369] mode=indexing
          w365 = refnum<k20> refnum  # Array I8
          n98 = Dynamic FPGA Interface Cast(Session In=w365, Type=w369) -> (Session Out=w370:refnum<k20>)
          n99 = xnode "Read/Write Control"("FPGA VI Reference In"=w370, "error in"=w367) -> ("error out"=w368:errorcluster, "Value"=w366:i8[])  [unwired: 1 out]
          n100 = call-poly <vilib>:"write data element.vi"("value"=w366, "index"=w371, "data table in"=w373) -> ("data table out"=w372:T1)  [unwired: 8 in]
        }
      }
      frame "Array of U64" {
        n101 = for {
          tunnel: w377 -> [w386] mode=indexing
          shift-right: [w383] -> w375
          shift-left: w376 -> [w382]
          shift-right: [w387] -> w378
          shift-left: w379 -> [w388]
          tunnel: w374 -> [w384] mode=indexing
          n102 = Dynamic FPGA Interface Cast(Session In=refnum<k20> refnum ("FPGA VI Reference Out"), Type=w384) -> (Session Out=w385:refnum<k20>)
          n103 = xnode "Read/Write Control"("FPGA VI Reference In"=w385, "error in"=w382) -> ("error out"=w383:errorcluster, "Value"=w381:u64[])  [unwired: 1 out]
          n104 = call-poly <vilib>:"write data element.vi"("value"=w381, "index"=w386, "data table in"=w388) -> ("data table out"=w387:T1)  [unwired: 8 in]
        }
      }
      frame "Array of U32" {
        n105 = for {
          tunnel: w392 -> [w401] mode=indexing
          shift-right: [w398] -> w390
          shift-left: w391 -> [w397]
          shift-right: [w402] -> w393
          shift-left: w394 -> [w403]
          tunnel: w389 -> [w399] mode=indexing
          w395 = refnum<k20> refnum  # Array U32
          n106 = Dynamic FPGA Interface Cast(Session In=w395, Type=w399) -> (Session Out=w400:refnum<k20>)
          n107 = xnode "Read/Write Control"("FPGA VI Reference In"=w400, "error in"=w397) -> ("error out"=w398:errorcluster, "Value"=w396:u32[])  [unwired: 1 out]
          n108 = call-poly <vilib>:"write data element.vi"("value"=w396, "index"=w401, "data table in"=w403) -> ("data table out"=w402:T1)  [unwired: 8 in]
        }
      }
      frame "Array of U16" {
        n109 = for {
          tunnel: w407 -> [w416] mode=indexing
          shift-right: [w413] -> w405
          shift-left: w406 -> [w412]
          shift-right: [w417] -> w408
          shift-left: w409 -> [w418]
          tunnel: w404 -> [w414] mode=indexing
          w410 = refnum<k20> refnum  # Array U16
          n110 = Dynamic FPGA Interface Cast(Session In=w410, Type=w414) -> (Session Out=w415:refnum<k20>)
          n111 = xnode "Read/Write Control"("FPGA VI Reference In"=w415, "error in"=w412) -> ("error out"=w413:errorcluster, "Value"=w411:u16[])  [unwired: 1 out]
          n112 = call-poly <vilib>:"write data element.vi"("value"=w411, "index"=w416, "data table in"=w418) -> ("data table out"=w417:T1)  [unwired: 8 in]
        }
      }
      frame "Array of U8" {
        n113 = for {
          tunnel: w422 -> [w431] mode=indexing
          shift-right: [w428] -> w420
          shift-left: w421 -> [w427]
          shift-right: [w432] -> w423
          shift-left: w424 -> [w433]
          tunnel: w419 -> [w429] mode=indexing
          w425 = refnum<k20> refnum  # Array U8
          n114 = Dynamic FPGA Interface Cast(Session In=w425, Type=w429) -> (Session Out=w430:refnum<k20>)
          n115 = xnode "Read/Write Control"("FPGA VI Reference In"=w430, "error in"=w427) -> ("error out"=w428:errorcluster, "Value"=w426:u8[])  [unwired: 1 out]
          n116 = call-poly <vilib>:"write data element.vi"("value"=w426, "index"=w431, "data table in"=w433) -> ("data table out"=w432:T1)  [unwired: 8 in]
        }
      }
      frame "Array of Boolean" {
        n117 = for {
          tunnel: w437 -> [w446] mode=indexing
          shift-right: [w443] -> w435
          shift-left: w436 -> [w442]
          shift-right: [w447] -> w438
          shift-left: w439 -> [w448]
          tunnel: w434 -> [w444] mode=indexing
          w440 = refnum<k20> refnum  # Array Boolean
          n118 = Dynamic FPGA Interface Cast(Session In=w440, Type=w444) -> (Session Out=w445:refnum<k20>)
          n119 = xnode "Read/Write Control"("FPGA VI Reference In"=w445, "error in"=w442) -> ("error out"=w443:errorcluster, "Value"=w441:bool[])  [unwired: 1 out]
          n120 = call-poly <vilib>:"write data element.vi"("value"=w441, "index"=w446, "data table in"=w448) -> ("data table out"=w447:T1)  [unwired: 8 in]
        }
      }
    }
  }
  "error out" <- w4
  "data table out" <- w3
  "io runtime out" <- "io runtime in"
